vi "Assign10Samples.vi"(6 "Last laser bit in":bool, 8 "PMT bits in":bool[](array[boolean])=[FALSE, FALSE, FALSE, FALSE, FALSE, FALSE, FALSE, FALSE, FALSE, FALSE], 9 "Laser bits in":bool[](array[boolean])=[FALSE, FALSE, FALSE, FALSE, FALSE, FALSE, FALSE, FALSE, FALSE, FALSE], 10 "Photon counters in":T1=[0, 0], 11 "Current region in":T2) -> (2 "Photon counters out":T1, 3 "Current region out":T2 max=1, 4 "Last laser bit out":bool)   [LabVIEW 2012]
uses:
  RegionalPhotonCounters.ctl
  RegionSelector.ctl
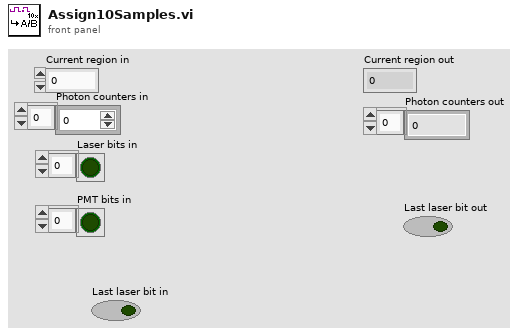
[diagram p1: front panel]
types:
  T1 = typedef "RegionalPhotonCounters.ctl" = i16[]
  T2 = typedef "RegionSelector.ctl" = i16
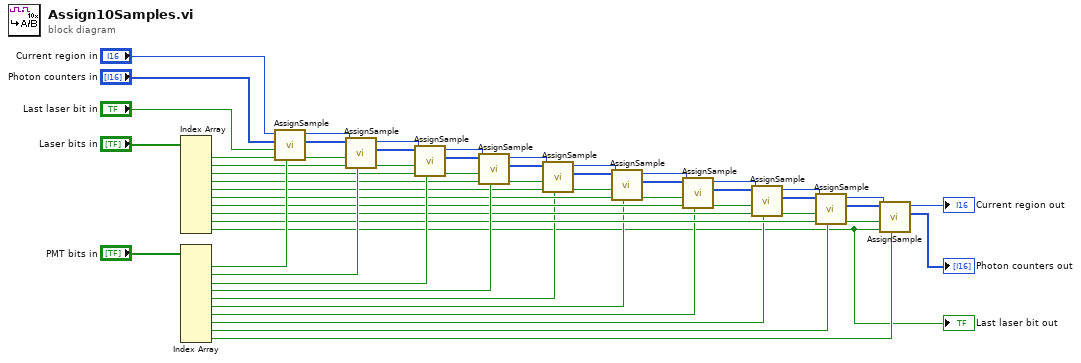
[diagram p0: block diagram]
diagram:
  n1 = Index Array(array="Laser bits in") -> (element #1=w37:bool, element #2=w33:bool, element #3=w29:bool, element #4=w25:bool, element #5=w14:bool, element #6=w13:bool, element #7=w12:bool, element #8=w11:bool, element #9=w10:bool, element #10=w1:bool)  [unwired: 10 in]
  "Last laser bit out" <- w1
  n2 = Index Array(array="PMT bits in") -> (element #1=w40:bool, element #2=w36:bool, element #3=w32:bool, element #4=w28:bool, element #5=w9:bool, element #6=w8:bool, element #7=w7:bool, element #8=w6:bool, element #9=w5:bool, element #10=w4:bool)  [unwired: 10 in]
  n3 = call "AssignSample.vi"("PMT state"=w40, "Current laser state"=w37, "Previous laser state"="Last laser bit in", "Photon counters in"="Photon counters in", "Region selector in"="Current region in") -> ("Photon counters out"=w38:T1, "Region selector out"=w39:T2)  [unwired: 5 in]
  n4 = call "AssignSample.vi"("PMT state"=w36, "Current laser state"=w33, "Previous laser state"=w37, "Photon counters in"=w38, "Region selector in"=w39) -> ("Photon counters out"=w34:T1, "Region selector out"=w35:T2)  [unwired: 5 in]
  n5 = call "AssignSample.vi"("PMT state"=w32, "Current laser state"=w29, "Previous laser state"=w33, "Photon counters in"=w34, "Region selector in"=w35) -> ("Photon counters out"=w30:T1, "Region selector out"=w31:T2)  [unwired: 5 in]
  n6 = call "AssignSample.vi"("PMT state"=w28, "Current laser state"=w25, "Previous laser state"=w29, "Photon counters in"=w30, "Region selector in"=w31) -> ("Photon counters out"=w26:T1, "Region selector out"=w27:T2)  [unwired: 5 in]
  n7 = call "AssignSample.vi"("PMT state"=w9, "Current laser state"=w14, "Previous laser state"=w25, "Photon counters in"=w26, "Region selector in"=w27) -> ("Photon counters out"=w15:T1, "Region selector out"=w16:T2)  [unwired: 5 in]
  n8 = call "AssignSample.vi"("PMT state"=w8, "Current laser state"=w13, "Previous laser state"=w14, "Photon counters in"=w15, "Region selector in"=w16) -> ("Photon counters out"=w23:T1, "Region selector out"=w24:T2)  [unwired: 5 in]
  n9 = call "AssignSample.vi"("PMT state"=w7, "Current laser state"=w12, "Previous laser state"=w13, "Photon counters in"=w23, "Region selector in"=w24) -> ("Photon counters out"=w21:T1, "Region selector out"=w22:T2)  [unwired: 5 in]
  n10 = call "AssignSample.vi"("PMT state"=w6, "Current laser state"=w11, "Previous laser state"=w12, "Photon counters in"=w21, "Region selector in"=w22) -> ("Photon counters out"=w19:T1, "Region selector out"=w20:T2)  [unwired: 5 in]
  n11 = call "AssignSample.vi"("PMT state"=w5, "Current laser state"=w10, "Previous laser state"=w11, "Photon counters in"=w19, "Region selector in"=w20) -> ("Photon counters out"=w17:T1, "Region selector out"=w18:T2)  [unwired: 5 in]
  n12 = call "AssignSample.vi"("PMT state"=w4, "Current laser state"=w1, "Previous laser state"=w10, "Photon counters in"=w17, "Region selector in"=w18) -> ("Photon counters out"=→"Photon counters out":T1, "Region selector out"=→"Current region out":T2)  [unwired: 5 in]
